vi "BSA_setup_check.vi"() -> (0 "ok":bool)   [LabVIEW 2010]
uses:
  Globals/LDA_meas_global_2.vi
  Globals/LDA_meas_global_1.vi
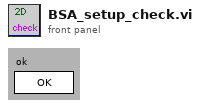
[diagram p1: front panel]
types:
  T1 = cluster{"Arrival time clock":enum16{"External", "Internal"}, "Clock source":enum16{"Slave", "Master", "Private"}, "Coincidence":enum16{"Slave", "Master", "Private"}}
  T2 = cluster{"Output data format":enum16{"Velocity, transit time, arrival time", "Velocity, arrival time", "Velocity, transit time", "Velocity"}, "Non-validated signals":enum16{"Accept", "Reject"}}
  T3 = enum16{"Velocity, transit time, arrival time", "Velocity, arrival time", "Velocity, transit time", "Velocity"}
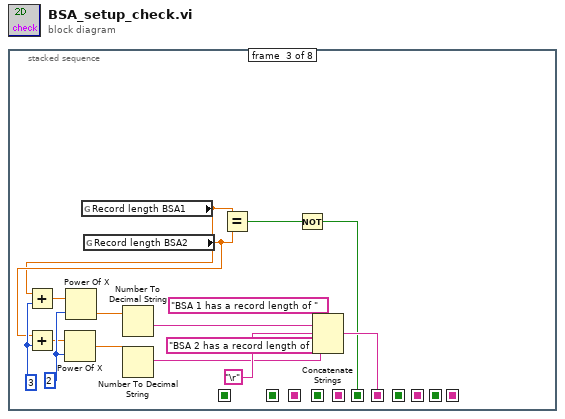
[diagram p0: block diagram]
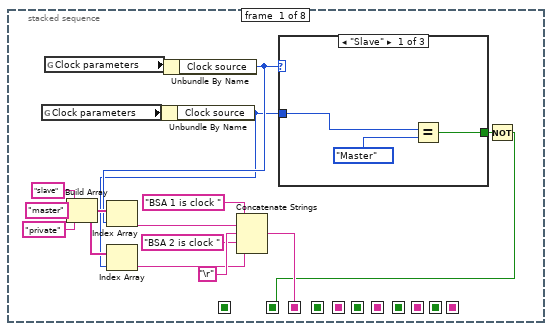
[diagram p2: hidden frame]
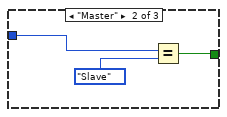
[diagram p3: hidden frame]
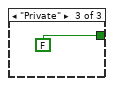
[diagram p4: hidden frame]
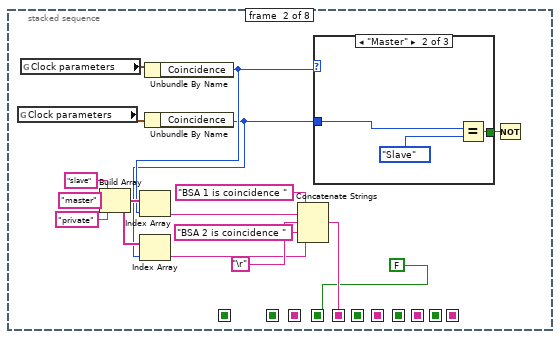
[diagram p5: hidden frame]
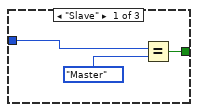
[diagram p6: hidden frame]
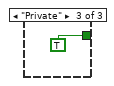
[diagram p7: hidden frame]
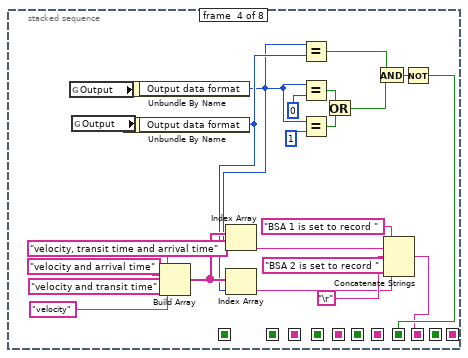
[diagram p8: hidden frame]
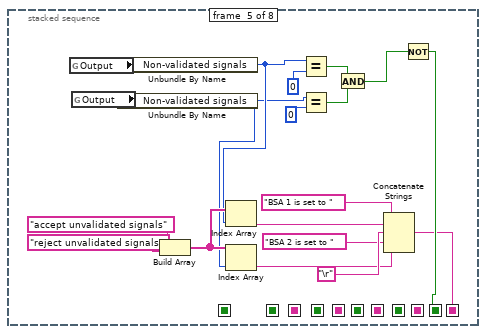
[diagram p9: hidden frame]
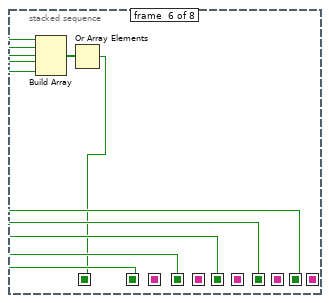
[diagram p10: hidden frame]
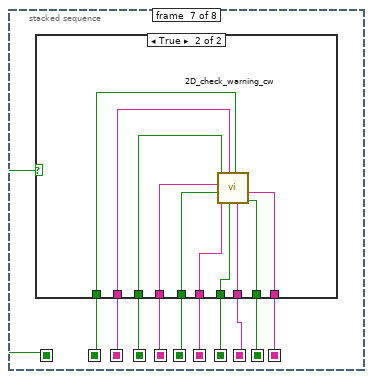
[diagram p11: hidden frame]
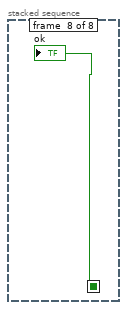
[diagram p13: hidden frame]
diagram:
  n1 = stacked-sequence {
    seq-local: [w3 _ _ _ _ _ _ _] -> [_ _ _ _ _ _ w121 _]
    seq-local: [w1 _ _ _ _ _ _ _] -> [_ _ _ _ _ w111 w122 _]
    seq-local: [_ FALSE _ _ _ _ _ _] -> [_ _ _ _ _ w110 w120 _]
    seq-local: [_ w28 _ _ _ _ _ _] -> [_ _ _ _ _ _ w119 _]
    seq-local: [_ _ w47 _ _ _ _ _] -> [_ _ _ _ _ w109 w118 _]
    seq-local: [_ _ w49 _ _ _ _ _] -> [_ _ _ _ _ _ w117 _]
    seq-local: [_ _ _ w64 _ _ _ _] -> [_ _ _ _ _ w108 w115 _]
    seq-local: [_ _ _ w63 _ _ _ _] -> [_ _ _ _ _ _ w116 _]
    seq-local: [_ _ _ _ _ w105 _ _] -> [_ _ _ _ _ _ w114 w133]
    seq-local: [_ _ _ _ w87 _ _ _] -> [_ _ _ _ _ w107 w113 _]
    seq-local: [_ _ _ _ w86 _ _ _] -> [_ _ _ _ _ _ w112 _]
    frame #0 {
      n2 = global read "LDA_meas_global_2.vi" "Clock parameters"() -> (w15:T1)
      n3 = global read "LDA_meas_global_1.vi" "Clock parameters"() -> (w16:T1)
      n4 = Build Array("slave", "master", "private") -> (w11:string[])
      n5 = Unbundle By Name(w15) -> ("Clock source"=w9:enum16{"Slave", "Master", "Private"})
      n6 = Index Array(array=w11, index=w9) -> (element=w4:string)
      n7 = Unbundle By Name(w16) -> ("Clock source"=w10:enum16{"Slave", "Master", "Private"})
      n8 = Index Array(array=w11, index=w10) -> (element=w7:string)
      n9 = Concatenate Strings("BSA 1 is clock ", w7, "\r", "BSA 2 is clock ", w4) -> (w3:string)
      n10 = case shown="\"Slave\"" w10 {
        tunnel: w9 -> [w18 w21 _]
        tunnel: [w17 w20 FALSE] -> w2
        frame "Slave" {
          n11 = Equal?(x=w18, y=enum16{"Slave", "Master", "Private"}."Master") -> (x = y?=w17:bool)
        }
        frame "Master" {
          n12 = Equal?(x=w21, y=enum16{"Slave", "Master", "Private"}."Slave") -> (x = y?=w20:bool)
        }
        frame "Private" {
        }
      }
      n13 = Not(x=w2) -> (.not. x?=w1:bool)
    }
    frame #1 {
      n14 = global read "LDA_meas_global_2.vi" "Clock parameters"() -> (w38:T1)
      n15 = global read "LDA_meas_global_1.vi" "Clock parameters"() -> (w39:T1)
      n16 = Build Array("slave", "master", "private") -> (w34:string[])
      n17 = Unbundle By Name(w39) -> ("Coincidence"=w27:enum16{"Slave", "Master", "Private"})
      n18 = Index Array(array=w34, index=w27) -> (element=w32:string)
      n19 = Unbundle By Name(w38) -> ("Coincidence"=w26:enum16{"Slave", "Master", "Private"})
      n20 = Index Array(array=w34, index=w26) -> (element=w29:string)
      n21 = Concatenate Strings("BSA 1 is coincidence ", w32, "\r", "BSA 2 is coincidence ", w29) -> (w28:string)
      n22 = case shown="\"Master\"" w27 {
        tunnel: w26 -> [w41 w44 _]
        tunnel: [w40 w43 TRUE] -> w25
        frame "Slave" {
          n23 = Equal?(x=w41, y=enum16{"Slave", "Master", "Private"}."Master") -> (x = y?=w40:bool)
        }
        frame "Master" {
          n24 = Equal?(x=w44, y=enum16{"Slave", "Master", "Private"}."Slave") -> (x = y?=w43:bool)
        }
        frame "Private" {
        }
      }
      n25 = Not(x=w25) -> ()  [unwired: 1 out]
    }
    frame #2 {
      w56 = 3
      w57 = 2
      n26 = global read "LDA_meas_global_1.vi" "Record length BSA1"() -> (w54:dbl)
      n27 = Add(x=w54, y=w56) -> (x+y=w51:dbl)
      n28 = Power Of X(1:w57, 2:w51) -> (0:w53:dbl)
      n29 = global read "LDA_meas_global_2.vi" "Record length BSA2"() -> (w55:dbl)
      n30 = Add(x=w55, y=w56) -> (x+y=w50:dbl)
      n31 = Power Of X(1:w57, 2:w50) -> (0:w52:dbl)
      n32 = Number To Decimal String(number=w53) -> (decimal integer string=w59:string)  [unwired: 1 out]
      n33 = Number To Decimal String(number=w52) -> (decimal integer string=w58:string)  [unwired: 1 out]
      n34 = Equal?(x=w54, y=w55) -> (x = y?=w62:bool)
      n35 = Not(x=w62) -> (.not. x?=w47:bool)
      n36 = Concatenate Strings("BSA 1 has a record length of ", w59, "\r", "BSA 2 has a record length of ", w58) -> (w49:string)
    }
    frame #3 {
      n37 = global read "LDA_meas_global_1.vi" "Output"() -> (w85:T2)
      n38 = global read "LDA_meas_global_2.vi" "Output"() -> (w84:T2)
      n39 = Unbundle By Name(w85) -> ("Output data format"=w72:T3)
      n40 = Unbundle By Name(w84) -> ("Output data format"=w73:T3)
      n41 = Build Array("velocity, transit time and arrival time", "velocity and arrival time", "velocity and transit time", "velocity") -> (w74:string[])
      n42 = Index Array(array=w74, index=w72) -> (element=w75:string)
      n43 = Index Array(array=w74, index=w73) -> (element=w77:string)
      n44 = Equal?(x=w72, y=w73) -> (x = y?=w66:bool)
      n45 = Equal?(x=w72, y=0) -> (x = y?=w69:bool)
      n46 = Equal?(x=w72, y=1) -> (x = y?=w68:bool)
      n47 = Or(x=w69, y=w68) -> (x .or. y?=w67:bool)
      n48 = And(x=w66, y=w67) -> (x .and. y?=w65:bool)
      n49 = Concatenate Strings("BSA 1 is set to record ", w75, "\r", "BSA 2 is set to record ", w77) -> (w63:string)
      n50 = Not(x=w65) -> (.not. x?=w64:bool)
    }
    frame #4 {
      n51 = global read "LDA_meas_global_1.vi" "Output"() -> (w104:T2)
      n52 = global read "LDA_meas_global_2.vi" "Output"() -> (w103:T2)
      n53 = Unbundle By Name(w104) -> ("Non-validated signals"=w91:enum16{"Accept", "Reject"})
      n54 = Unbundle By Name(w103) -> ("Non-validated signals"=w90:enum16{"Accept", "Reject"})
      n55 = Build Array("accept unvalidated signals", "reject unvalidated signals") -> (w95:string[])
      n56 = Index Array(array=w95, index=w91) -> (element=w96:string)
      n57 = Index Array(array=w95, index=w90) -> (element=w98:string)
      n58 = Equal?(x=w91, y=0) -> (x = y?=w89:bool)
      n59 = Equal?(x=w90, y=0) -> (x = y?=w88:bool)
      n60 = And(x=w89, y=w88) -> (x .and. y?=w92:bool)
      n61 = Concatenate Strings("BSA 1 is set to ", w96, "\r", "BSA 2 is set to ", w98) -> (w86:string)
      n62 = Not(x=w92) -> (.not. x?=w87:bool)
    }
    frame #5 {
      n63 = Build Array(w111, w110, w109, w108, w107) -> (w106:bool[])
      n64 = Or Array Elements(Boolean array=w106) -> (logical OR=w105:bool)
    }
    frame #6 {
      n65 = case shown="True" w114 {
        tunnel: w115 -> [_ w132]
        tunnel: w116 -> [_ w131]
        tunnel: w117 -> [_ w130]
        tunnel: w118 -> [_ w129]
        tunnel: w119 -> [_ w128]
        tunnel: w120 -> [_ w127]
        tunnel: w121 -> [_ w126]
        tunnel: w122 -> [_ w125]
        tunnel: w113 -> [_ w124]
        tunnel: w112 -> [_ w123]
        frame False {
        }
        frame True {
          n66 = call "2D_check_warning_cw.vi"("val"=w124, "validated"=w123, "data type"=w131, "at"=w125, "dt"=w132, "arr time clock"=w126, "record interval"=w130, "ri"=w129, "coincidence"=w128, "co"=w127) -> ()  [unwired: 1 in, 1 out]
        }
      }
    }
    frame #7 {
      "ok" <- w133
    }
  }
